vi "fast calibration..vi"() -> ()   [LabVIEW 2016]
uses:
  <vilib>/vision/Measure.llb/Edge Options.ctl
  <vilib>/vision/Measure.llb/Edge Polarity.ctl
  <vilib>/Analysis/6fits.llb/Curve Fitting Criteria.ctl
  <vilib>/Utility/file.llb/Read Delimited Spreadsheet (DBL).vi
  <vilib>/vision/NI_Vision_Development_Module.lvlib
  <resource>/objmgr/IMAQImage.rc
  <vilib>/Analysis/NI_AALBase.lvlib
  <vilib>/Analysis/NI_AALPro.lvlib
panel:
  out "decimated array 2":dbl[](array[numeric])
  out "decimated array":dbl[](array[numeric])
  in  "method":T1 items=["Least Square", "Least Absolute Residual", "Bisquare"]
  in  "Tab Control":T2(tab)
  in  "Coordinate Path.":path
  in  "Template Path":path
  in  "Image Path":path
  out "Y pixel":dbl
  out "X pixel":dbl
  out "coordinates":dbl[][](array[numeric])
  out "angle.":dbl
  out "angle in radian.":dbl
  out "Mean":dbl[][](array[numeric])
  out "standard deviation":dbl[][](array[numeric])
  out "ratio of good position.":dbl[](array[numeric])
  in  "Settings":T3={"Algorithm"=1, "Number of Matches Requested"=1, "Minimum Match Score"=800.0, "SubPixel Accuracy"=TRUE, "Rotation Angle Ranges"=[{"Start"=0.0, "End"=360.0}], "Show Search Area"=FALSE, "Show Result"=TRUE} {"Rotation Angle Ranges"."End" format="%.1f"; "Rotation Angle Ranges"."Start" format="%.1f"; "Minimum Match Score" min=0 max=1000 format="%.2f"; "Number of Matches Requested" min=1; "Algorithm" items=["All", "Low Discrepancy Sampling", "Grayscale Value Pyramid", "Gradients Pyramid"]}
  in  "Circle Fit Options":T4={"Process"=enum."Get First Edge", "Step Size"=3.0, "Max Pixel Radius"=3}
  in  "Options":T7={"Search  Direction"=1, "Edge Options"={"Edge Polarity"=0, "Kernel Size"=3, "Width"=3, "Minimum Edge Strength"=10.0, "Interpolation Type"=enum."Bilinear Fixed", "Data Processing Method"=enum."Average"}, "Show Search Area"=FALSE, "Show Search Lines"=FALSE, "Show Edges Found"=FALSE, "Show Result"=TRUE, "Search Area Color"=65280, "Search Lines Color"=255, "Edge Locations Color"=16776960, "Result Color"=16711680, "Overlay Group Name"=""} {"Search  Direction" items=["Outside to Inside", "Inside to Outside"]; "Edge Options"."Edge Polarity" items=["All Edges", "Rising Edges", "Falling Edges"]; "Edge Options"."Minimum Edge Strength" format="%.2f"; "Edge Options"."Width" step=2; "Edge Options"."Kernel Size" step=2}
  in  "Annulus ROI Descriptor":T8={"Global Rectangle"=[675, 567, 1751, 1642], "Contours"=[{"ID"=enum."External", "Type"=7, "Coordinates"=[1212, 1104, 85, 537, 0, 0]}]} {"Contours"."Type" items=["No Selection", "Point", "Line", "Rectangle", "Oval", "Polygon", "Freehand Region", "Annulus", "Unused2", "Unused3", "Broken Line", "Freehand Line", "Rotated Rectangle"]}
  out "Fitted Circle":T9 {"Average SNR (dB)" format="%.2f"; "Average Strength" format="%.2f"; "Roundness (Real-World)" format="%.2f"; "Radius (Real-World)" format="%.2f"; "Center (Real-World)"."Y" format="%.2f"; "Center (Real-World)"."X" format="%.2f"; "Radius (Pixels)" format="%.2f"; "Center (Pixels)"."Y" format="%.2f"; "Center (Pixels)"."X" format="%.2f"}
  out "Resulting ROI":T10
  out "Array":T11[](array[plugin-control])
  in  "No of each images":dbl
  in  "No of pin":dbl=7.0
  in  "Pixel to micron":dbl=1.58
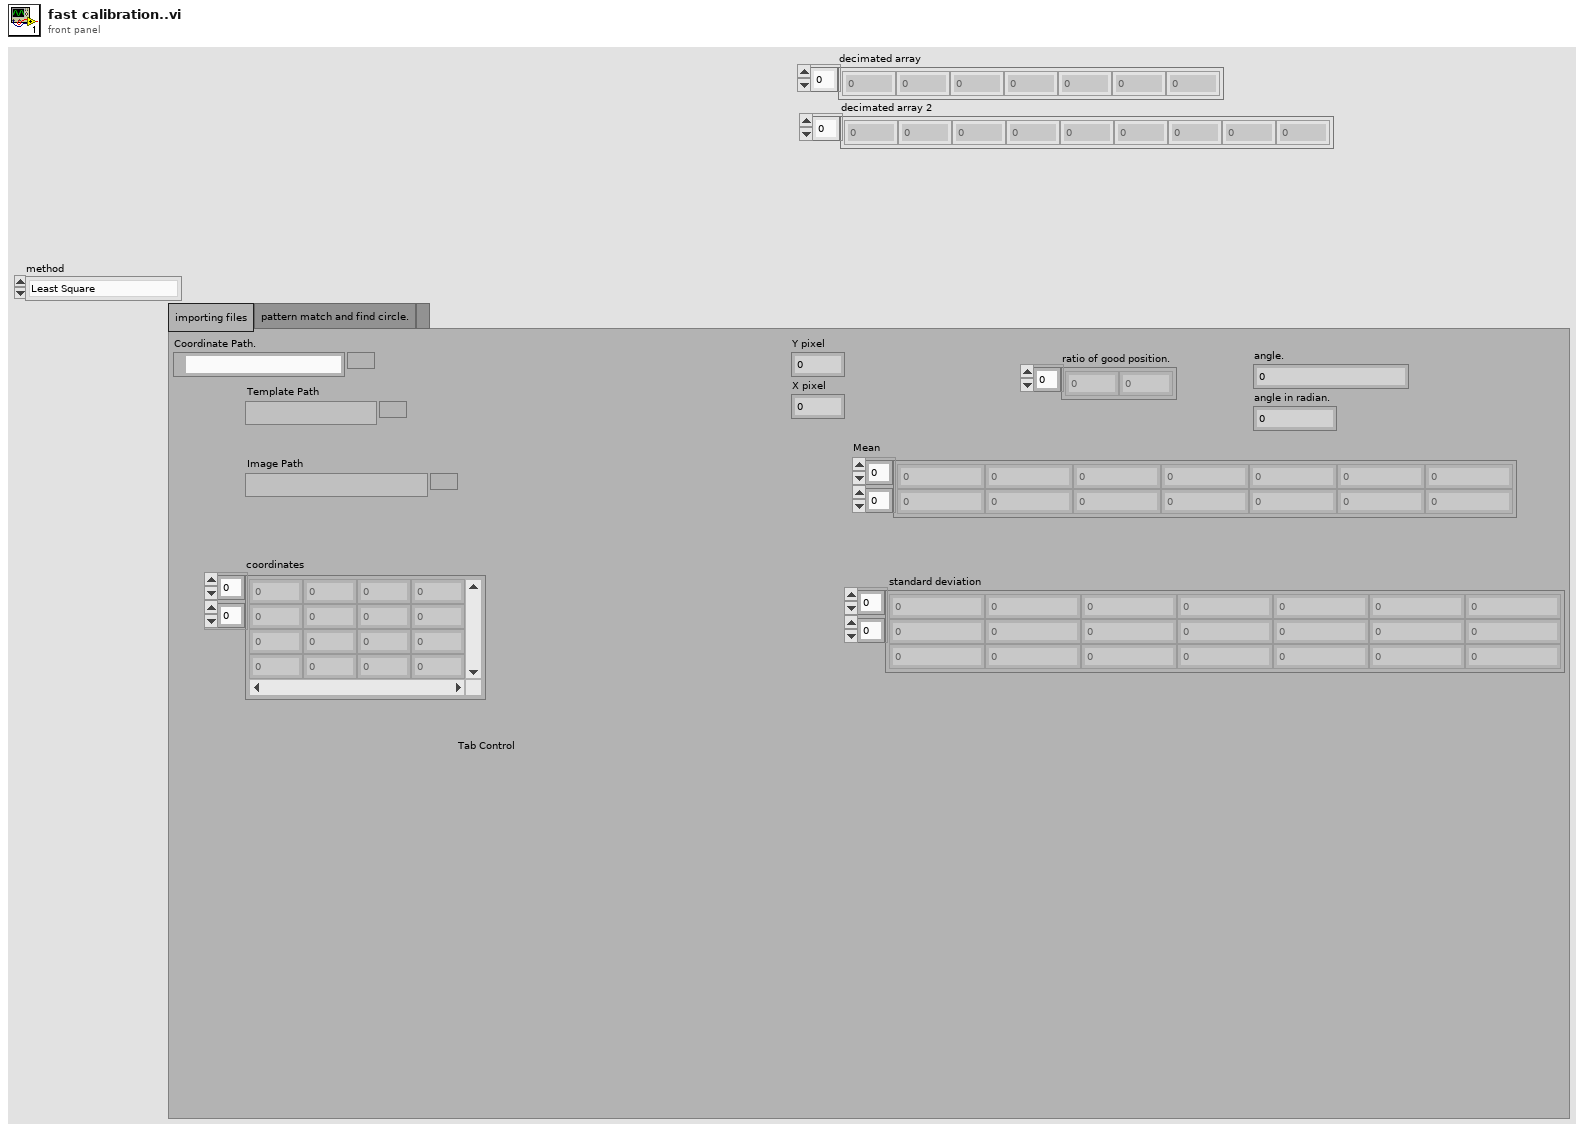
[diagram p1: front panel]
types:
  T1 = typedef "NI_AALPro.lvlib/Curve Fitting Criteria.ctl" = u16
  T2 = enum32{"importing files", "pattern match and find circle.", ""}
  T3 = cluster{"Algorithm":i32, "Number of Matches Requested":i32, "Minimum Match Score":sgl, "SubPixel Accuracy":bool, "Rotation Angle Ranges":cluster{"Start":sgl, "End":sgl}[], "Show Search Area":bool, "Show Result":bool}
  T4 = cluster{"Process":enum16{"Get First Edge", "Get First + Last Edge", "Get All Edges", "Get Best Edge"}, "Step Size":dbl, "Max Pixel Radius":i32}
  T5 = typedef "Edge Options.ctl" = cluster{"Edge Polarity":T6, "Kernel Size":u32, "Width":u32, "Minimum Edge Strength":sgl, "Interpolation Type":enum32{"Zero Order", "Bilinear", "Quadratic", "Cubic", "Bilinear Fixed"}, "Data Processing Method":enum32{"Average", "Median"}}
  T6 = typedef "Edge Polarity.ctl" = u32
  T7 = cluster{"Search  Direction":u32, "Edge Options":T5, "Show Search Area":bool, "Show Search Lines":bool, "Show Edges Found":bool, "Show Result":bool, "Search Area Color":u32, "Search Lines Color":u32, "Edge Locations Color":u32, "Result Color":u32, "Overlay Group Name":string}
  T8 = cluster{"Global Rectangle":i32[], "Contours":cluster{"ID":enum32{"External", "Internal"}, "Type":u32, "Coordinates":i32[]}[]}
  T9 = cluster{"Center (Pixels)":cluster{"X":sgl, "Y":sgl}, "Radius (Pixels)":dbl, "Center (Real-World)":cluster{"X":sgl, "Y":sgl}, "Radius (Real-World)":dbl, "Roundness (Real-World)":dbl, "Average Strength":dbl, "Average SNR (dB)":dbl}
  T10 = cluster{sgl[], cluster{"ID":enum32{"External", "Internal"}, "Type":u32, "Coordinates":i32[]}[]}
  T11 = typedef "IMAQ Image.ctl" = refnum<image>
  T12 = cluster{"ID":enum32{"External", "Internal"}, "Type":u32, "Coordinates":i32[]}[]
  T13 = cluster{"Position":cluster{"x":sgl, "y":sgl}, "Angle":sgl, "Scale":sgl, "Score":sgl, "Bounding Box":cluster{"x":sgl, "y":sgl}[]}[]
  T14 = cluster{"ID":enum32{"External", "Internal"}, "Type":u32, "Coordinates":i32[]}
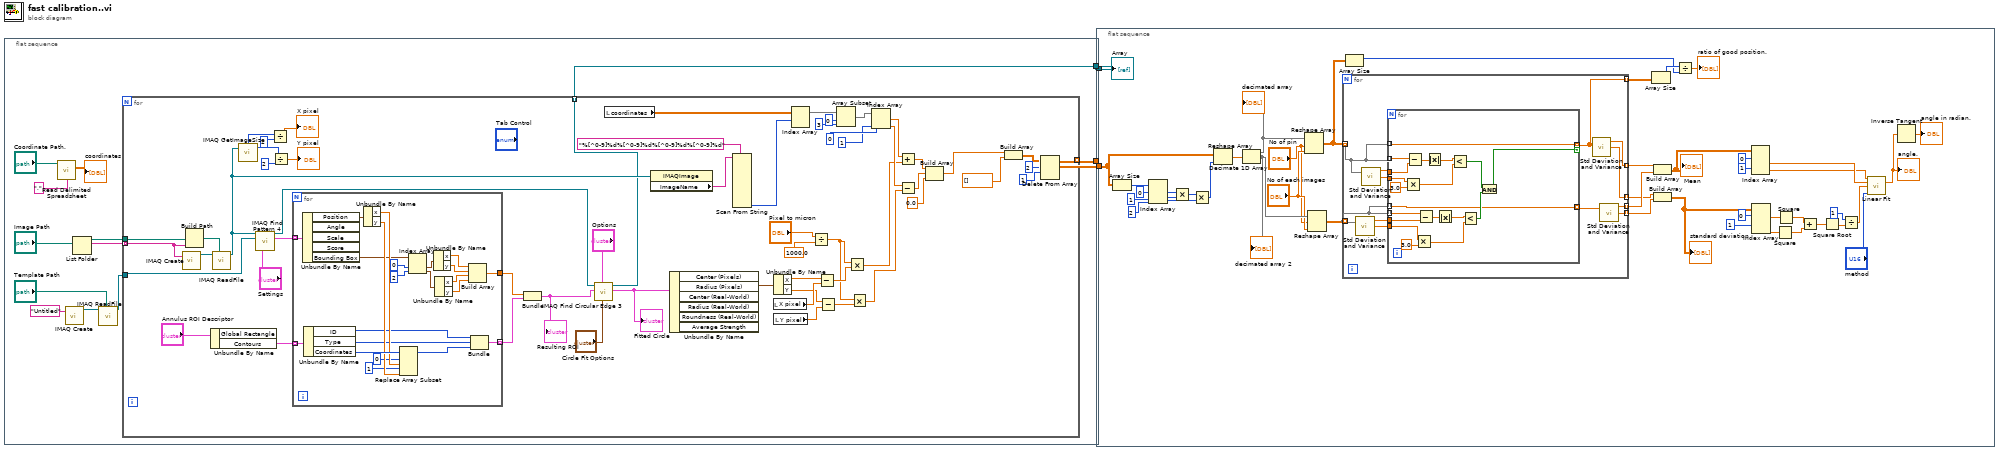
[diagram p0: block diagram]
diagram:
  n1 = flat-sequence {
    tunnel: [w3] -> w2
    tunnel: [w4] -> w1
    frame #0 {
      n2 = call-poly <vilib>:"Read Delimited Spreadsheet.vi"("file path (dialog if empty)"="Coordinate Path.", "delimiter (\\t)"="," ("delimiter (\\t)")) -> ("all rows"=→"coordinates":dbl[][])  [unwired: 8 in, 5 out]
      n3 = call "IMAQ Create"("Image Name"="Untitled") -> ("New Image"=w14:T11)  [unwired: 4 in, 1 out]
      n4 = List Folder(path="Image Path") -> (path out=w9:path, filenames=w10:string[])  [unwired: 3 in, 2 out]
      n5 = call "IMAQ ReadFile"("File Path"="Template Path", "Image"=w14) -> ("Image Out"=w8:T11)  [unwired: 5 in, 4 out]
      n6 = for {
        tunnel: w10 -> [w69] mode=indexing
        tunnel: w9 -> [w66]
        tunnel: w8 -> [w68]
        tunnel: [w40] -> w3 mode=indexing
        tunnel: [w29] -> w4 mode=indexing
        n7 = call "IMAQ Create"("Image Name"=w69) -> ("New Image"=w71:T11)  [unwired: 4 in, 1 out]
        n8 = Build Path(base path=w66, name or relative path=w69) -> (appended path=w70:path)
        n9 = Unbundle By Name("Annulus ROI Descriptor") -> ("Contours"=w63:T12)  [unwired: 1 out]
        n10 = call "IMAQ ReadFile"("File Path"=w70, "Image"=w71) -> ("Image Out"=w45:T11)  [unwired: 5 in, 4 out]
        n11 = call "IMAQ GetImageSize"("Image"=w45) -> ("Y Resolution"=w53:i32, "X Resolution"=w55:i32)  [unwired: 3 in, 1 out]
        n12 = call "IMAQ Find Pattern 4"("Image"=w45, "Template"=w68, "Settings"="Settings") -> ("Image Out"=w58:T11, "Matches (pixel)"=w65:T13)  [unwired: 6 in, 5 out]
        n13 = Divide(x=w55, y=2) -> (x/y=→"X pixel":dbl)
        n14 = Divide(x=w53, y=2) -> (x/y=→"Y pixel":dbl)
        n15 = for {
          tunnel: w65 -> [w93] mode=indexing
          tunnel: w63 -> [w91] mode=indexing
          tunnel: [w73] -> w62
          tunnel: [w72] -> w61 mode=indexing
          n16 = Unbundle By Name(w93) -> ("Position"=w92:cluster{"x":sgl, "y":sgl}, "Bounding Box"=w82:cluster{"x":sgl, "y":sgl}[])  [unwired: 3 out]
          n17 = Unbundle By Name(w91) -> ("ID"=w83:enum32{"External", "Internal"}, "Type"=w84:u32, "Coordinates"=w90:i32[])
          n18 = Unbundle By Name(w92) -> ("x"=w89:sgl, "y"=w88:sgl)
          n19 = Replace Array Subset(array=w90, new element #1=w89, index #1=0 ("index"), new element #2=w88, index #2=1 ("index")) -> (w85:i32[])
          n20 = Index Array(array=w82, index #1=0 ("index"), index #2=2 ("index")) -> (element #1=w78:cluster{"x":sgl, "y":sgl}, element #2=w79:cluster{"x":sgl, "y":sgl})
          n21 = Unbundle By Name(w78) -> ("x"=w74:sgl, "y"=w75:sgl)
          n22 = Unbundle By Name(w79) -> ("x"=w76:sgl, "y"=w77:sgl)
          n23 = Build Array(w74, w75, w76, w77) -> (w73:sgl[])
          n24 = Bundle("ID"=w83, "Type"=w84, "Coordinates"=w85) -> (w72:T14)  [unwired: 1 in]
        }
        n25 = Bundle(w62, w61) -> (w60:T10)  [unwired: 1 in]
        "Resulting ROI" <- w60
        n26 = call "IMAQ Find Circular Edge 3"("Circle Fit Options"="Circle Fit Options", "Options"="Options", "ROI Descriptor"=w60, "Image"=w58) -> ("Fitted Circle"=w57:T9, "Image Out"=w40:T11)  [unwired: 3 in, 3 out]
        "Fitted Circle" <- w57
        n27 = local read "coordinates"() -> (w42:dbl[][])
        n28 = property class="IMAQImage"(reference=w45) -> ("ImageName"=w44:string)  [unwired: 1 in, 2 out]
        n29 = Unbundle By Name(w57) -> ("Center (Pixels)"=w16:cluster{"X":sgl, "Y":sgl})  [unwired: 5 out]
        n30 = Scan From String(format string="%[^0-9]%d%[^0-9]%d%[^0-9]%d%[^0-9]%d", input string=w44) -> (output 8=w41:i32)  [unwired: 17 in, 3 out]
        n31 = local read "X pixel"() -> (w48:dbl)
        n32 = Unbundle By Name(w16) -> ("X"=w49:sgl, "Y"=w47:sgl)
        n33 = local read "Y pixel"() -> (w46:dbl)
        n34 = Index Array(array=w42, index (row)=w41) -> (element=w21:dbl[])  [unwired: 1 in]
        n35 = Divide(x="Pixel to micron", y=1000.0) -> (x/y=w33:dbl)
        n36 = Subtract(x=w49, y=w48) -> (x-y=w34:dbl)
        n37 = Subtract(x=w47, y=w46) -> (x-y=w35:dbl)
        n38 = Array Subset(array=w21, index=0, length=3) -> (w15:dbl[])
        n39 = Multiply(x=w33, y=w34) -> (x*y=w20:dbl)
        n40 = Multiply(x=w33, y=w35) -> (x*y=w19:dbl)
        n41 = Index Array(array=w15, index #1=0 ("index"), index #2=1 ("index")) -> (element #1=w24:dbl, element #2=w25:dbl)
        n42 = Add(x=w24, y=w20) -> (x+y=w28:dbl)
        n43 = Subtract(x=w25, y=w19) -> (x-y=w27:dbl)
        n44 = Build Array(w28, w27, 0.0 ("element")) -> (w26:dbl[])
        n45 = Build Array(w26, dbl[] [] ("element")) -> (w18:dbl[][])
        n46 = Delete From Array(array=w18, length=2, index (row)=1) -> (array with subset deleted=w29:dbl[][])  [unwired: 1 in, 1 out]
      }
    }
  }
  n47 = flat-sequence {
    tunnel: w2 -> [w138]
    tunnel: w1 -> [w129]
    frame #0 {
      n48 = Array Size(array=w129) -> (size(s)=w137:i32[])
      n49 = Index Array(array=w137, index #1=0 ("index"), index #2=1 ("index"), index #3=2 ("index")) -> (element #1=w133:i32, element #2=w132:i32, element #3=w130:i32)
      n50 = Multiply(x=w133, y=w132) -> (x*y=w131:i32)
      n51 = Multiply(x=w131, y=w130) -> (x*y=w128:i32)
      n52 = Reshape Array(w129, w128) -> (w127:dbl[])
      n53 = Decimate 1D Array(w127) -> (w126:dbl[], w125:dbl[])  [unwired: 1 out]
      "decimated array" <- w126
      "decimated array 2" <- w125
      n54 = Reshape Array(w126, "No of pin", "No of each images") -> (w119:dbl[][])
      n55 = Reshape Array(w125, "No of pin", "No of each images") -> (w120:dbl[][])
      n56 = for {
        tunnel: w120 -> [w139] mode=indexing
        tunnel: [w145] -> w104 mode=indexing
        tunnel: [w144] -> w122 mode=indexing
        tunnel: w119 -> [w140] mode=indexing
        tunnel: [w143] -> w94 mode=indexing
        tunnel: [w142] -> w118 mode=indexing
        tunnel: [w141] -> w95 mode=indexing
        n57 = call <vilib>:"Std Deviation and Variance.vi"("X"=w139) -> ("mean"=w148:dbl, "standard deviation"=w147:dbl)  [unwired: 1 in, 1 out]
        n58 = call <vilib>:"Std Deviation and Variance.vi"("X"=w140) -> ("mean"=w149:dbl, "standard deviation"=w150:dbl)  [unwired: 1 in, 1 out]
        n59 = for {
          tunnel: w140 -> [w155] mode=indexing
          tunnel: [w152] -> w144 mode=indexing if=w169
          tunnel: w150 -> [w168]
          tunnel: w149 -> [w166]
          tunnel: w139 -> [w154] mode=indexing
          tunnel: w148 -> [w158]
          tunnel: w147 -> [w157]
          tunnel: [w151] -> w146 mode=indexing
          tunnel: w140 -> [w152] mode=indexing
          tunnel: w139 -> [w151] mode=indexing
          n60 = Multiply(x=w168, y=3.0 ("x")) -> (x*y=w163:dbl)
          n61 = Subtract(x=w155, y=w166) -> (x-y=w165:dbl)
          n62 = Multiply(x=w157, y=3.0 ("x")) -> (x*y=w159:dbl)
          n63 = Subtract(x=w154, y=w158) -> (x-y=w161:dbl)
          n64 = Absolute Value(x=w165) -> (abs(x)=w164:dbl)
          n65 = Absolute Value(x=w161) -> (abs(x)=w160:dbl)
          n66 = Less?(x=w164, y=w163) -> (x < y?=w162:bool)
          n67 = Less?(x=w160, y=w159) -> (x < y?=w156:bool)
          n68 = And(x=w162, y=w156) -> (x .and. y?=w169:bool)
        }
        n69 = call <vilib>:"Std Deviation and Variance.vi"("X"=w144) -> ("mean"=w145:dbl, "standard deviation"=w143:dbl)  [unwired: 1 in, 1 out]
        n70 = call <vilib>:"Std Deviation and Variance.vi"("X"=w146) -> ("mean"=w141:dbl, "standard deviation"=w142:dbl)  [unwired: 1 in, 1 out]
      }
      n71 = Array Size(array=w119) -> (size(s)=w117:i32[])
      n72 = Array Size(array=w122) -> (size(s)=w121:i32[])
      n73 = Build Array(w104, w95) -> (w101:dbl[][])
      "Mean" <- w101
      n74 = Build Array(w94, w118) -> (w115:dbl[][])
      "standard deviation" <- w115
      n75 = Divide(x=w121, y=w117) -> (x/y=→"ratio of good position.":dbl[])
      n76 = Index Array(array=w101, index (row) #1=0 ("index (row)"), index (row) #2=1 ("index (row)")) -> (element #1=w98:dbl[], element #2=w97:dbl[])  [unwired: 2 in]
      n77 = Index Array(array=w115, index (row) #1=0 ("index (row)"), index (row) #2=1 ("index (row)")) -> (element #1=w111:dbl[], element #2=w112:dbl[])  [unwired: 2 in]
      n78 = Square(x=w112) -> (x^2=w110:dbl[])
      n79 = Square(x=w111) -> (x^2=w109:dbl[])
      n80 = Add(x=w109, y=w110) -> (x+y=w108:dbl[])
      n81 = Square Root(x=w108) -> (sqrt(x)=w107:dbl[])
      n82 = Divide(x=1, y=w107) -> (x/y=w105:dbl[])
      n83 = call <vilib>:"Linear Fit.vi"("Y"=w97, "X"=w98, "Weight"=w105, "method"="method") -> ("slope"=w103:dbl)  [unwired: 7 in, 4 out]
      "angle." <- w103
      n84 = Inverse Tangent(1:w103) -> (0:→"angle in radian.":dbl)
      "Array" <- w138
    }
  }
